vi "Do.vi"(8 "error in (no error)":errorcluster, 10 "FormulaG API":refnum<class "FormulaG API.lvclass">, 11 "Reset Cmd in":refnum<class "Reset Cmd.lvclass">) -> (0 "error out":errorcluster, 3 "Reset Cmd out":refnum<class "Reset Cmd.lvclass">)   [LabVIEW 2024, in "FormulaG.lvlib" / "Reset Cmd.lvclass"]
uses:
  Reset Cmd.lvclass
  FormulaG API/FormulaG API.lvclass
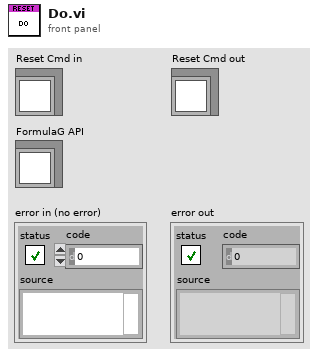
[diagram p1: front panel]
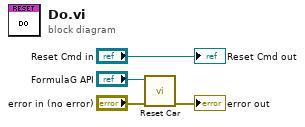
[diagram p0: block diagram]
diagram:
  n1 = call "Reset Car.vi"("error in (no error)"="error in (no error)", "FormulaG API in"="FormulaG API") -> ("error out"=→"error out":errorcluster)  [unwired: 8 in, 1 out]
  "Reset Cmd out" <- "Reset Cmd in"
